vi "Read File.vi"(8 "error in (no error)":errorcluster, 11 "[User] Userinfo Binary in":refnum<class "[User] Userinfo Binary.lvclass">) -> (0 "error out":errorcluster, 3 "[User] Userinfo Binary out":refnum<class "[User] Userinfo Binary.lvclass">)   [LabVIEW 2020, in "[User] Userinfo Binary.lvclass"]
uses:
  [User] Userinfo Binary.lvclass
  Control/userinfo.ctl
  [User] Userinfo Binary.lvclass/[User] Userinfo Binary.ctl
  <vilib>/YU/YU-Encrypt/AES/AES.lvclass
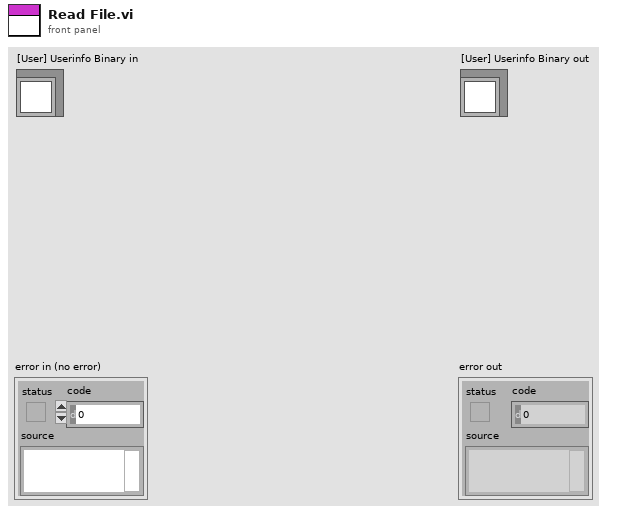
[diagram p1: front panel]
types:
  T1 = typedef "[User] Userinfo Binary.lvclass/userinfo.ctl" = cluster{"password":string, "authority":i8, "department":string, "post":string, "remark":string, "create time":timestamp, "last login time":timestamp}
  T2 = enum16{"open", "replace", "create", "open or create", "replace or create", "replace or create with confirmation"}
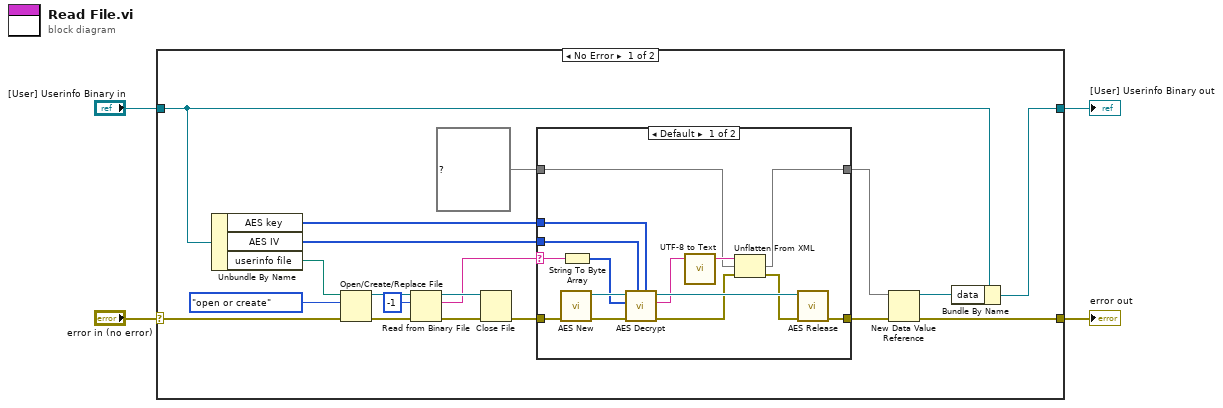
[diagram p0: block diagram]
diagram:
  n1 = case shown="No Error" "error in (no error)" {
    selector: "error in (no error)" -> [w23 w42]
    tunnel: [w9 w42] -> w1
    tunnel: [w12 w41] -> w2
    tunnel: "[User] Userinfo Binary in" -> [w13 w41]
    frame No Error {
      n2 = Unbundle By Name(w13) -> ("AES key"=w14:u8[], "AES IV"=w15:u8[], "userinfo file"=w22:path)
      n3 = Open/Create/Replace File(file path (use dialog)=w22, error in=w23, operation (0:open)=T2."open or create") -> (refnum out=w19:refnum<file>, error out=w20:errorcluster)  [unwired: 3 in, 1 out]
      n4 = Read from Binary File(8:w20, 10:-1 ("count (1)"), 11:w19) -> (0:w18:errorcluster, 2:w7:string, 3:w17:refnum<file>)  [unwired: 3 in, 1 out]
      n5 = Close File(refnum=w17, error in=w18) -> (error out=w16:errorcluster)  [unwired: 1 out]
      n6 = case shown="Default" w7 {
        selector: w7 -> [w24 _]
        tunnel: w16 -> [w34 w40]
        tunnel: [w32 w40] -> w11
        tunnel: w15 -> [w35 _]
        tunnel: w14 -> [w36 _]
        tunnel: map{string, T1} {} ("data") -> [w26 w39]
        tunnel: [w25 w39] -> w10
        frame Default {
          n7 = call <vilib>:"AES New.vi"("error in (no error)"=w34) -> ("error out"=w38:errorcluster, "AES out"=w37:refnum<class "AES.lvclass">)  [unwired: 9 in]
          n8 = String To Byte Array(string=w24) -> (unsigned byte array=w30:u8[])
          n9 = call <vilib>:"AES Decrypt.vi"("Key"=w36, "IV"=w35, "error in (no error)"=w38, "encrypted data"=w30, "AES in"=w37) -> ("error out"=w28:errorcluster, "data"=w31:string, "AES out"=w33:refnum<class "AES.lvclass">)  [unwired: 4 in]
          n10 = call <vilib>:"UTF-8 to Text.vi"("utf-8 text"=w31) -> ("text"=w29:string)  [unwired: 4 in]
          n11 = Unflatten From XML(xml string=w29, type=w26, error in (no error)=w28) -> (value=w25:map{string, T1}, error out=w27:errorcluster)
          n12 = call <vilib>:"AES Release.vi"("error in (no error)"=w27, "AES in"=w33) -> ("error out"=w32:errorcluster)  [unwired: 9 in]
        }
        frame "" {
        }
      }
      n13 = New Data Value Reference(data value=w10, error in=w11) -> (data value reference=w5:refnum<data-value>, error out=w9:errorcluster)
      n14 = Bundle By Name(cluster=w13, "data"=w5) -> (w12:refnum<class "[User] Userinfo Binary.lvclass">)
    }
    frame Error {
    }
  }
  "error out" <- w1
  "[User] Userinfo Binary out" <- w2
